vi "Update Tree.vi"(7 "Tree":refnum<vi>, 8 "error in (no error)":errorcluster, 10 "Task Run Info":T1[](array[typedef])) -> (0 "error out":errorcluster)   [LabVIEW 2020, in "Volatus.lvlib" / "DebugGUI.lvclass"]
uses:
  DebugGUI.lvclass
  Task Run Info.ctl
  Task Hierarchy.ctl
  Task State.ctl
  DebugGUI.lvclass/DebugGUI.ctl
  Volatus.lvlib
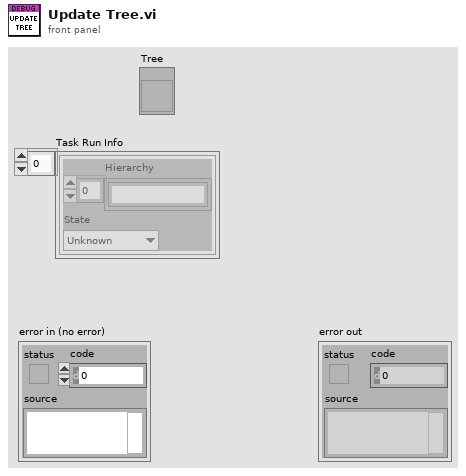
[diagram p1: front panel]
types:
  T1 = typedef "Volatus.lvlib/Task Run Info.ctl" = cluster{"Hierarchy":T2, "State":T3}
  T2 = typedef "Volatus.lvlib/Task Hierarchy.ctl" = string[]
  T3 = typedef "Volatus.lvlib/Task State.ctl" = enum16{"Unknown", "Idle", "Initializing", "Starting", "Running", "Stopping", "Stopped", "Error - Init", "Error - Start", "Error - Run", "Error - Stop"}
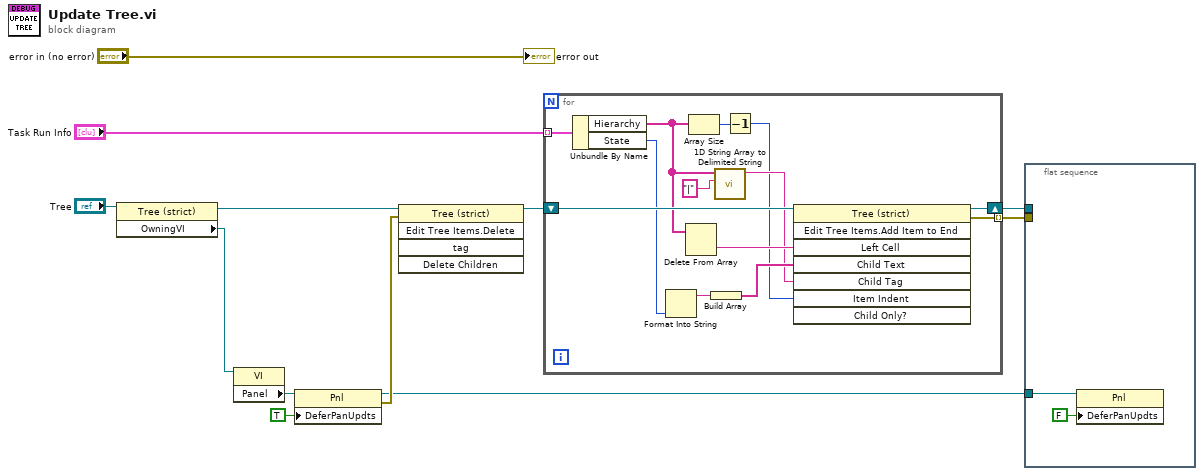
[diagram p0: block diagram]
diagram:
  n1 = property class="Tree (strict)"(reference="Tree") -> (reference out=w7:refnum<vi>, "OwningVI"=w10:refnum<vi>)  [unwired: 1 in, 1 out]
  n2 = property class="VI"(reference=w10) -> ("Panel"=w9:refnum<vi>)  [unwired: 1 in, 2 out]
  n3 = property class="Pnl"(reference=w9, "DeferPanUpdts"=TRUE ("Defer Panel Updates")) -> (reference out=w3:refnum<vi>, error out=w6:errorcluster)  [unwired: 1 in]
  n4 = invoke class="Tree (strict)" method="Edit Tree Items.Delete"(reference=w7, error in=w6) -> (reference out=w5:refnum<vi>)  [unwired: 3 in, 4 out]
  n5 = for {
    shift-right: [w15] -> w2
    shift-left: w5 -> [w25]
    tunnel: "Task Run Info" -> [w24] mode=indexing
    tunnel: [w14] -> w1 mode=indexing
    n6 = Unbundle By Name(w24) -> ("Hierarchy"=w18:T2, "State"=w23:T3)
    n7 = Format Into String(w23) -> (resulting string=w22:string)  [unwired: 3 in, 1 out]
    n8 = Delete From Array(array=w18) -> (deleted portion=w20:string)  [unwired: 2 in, 1 out]
    n9 = Array Size(array=w18) -> (size(s)=w19:i32)
    n10 = Build Array(w22) -> (w21:string[])
    n11 = call <vilib>:"1D String Array to Delimited String.vi"("delimiter"="|", "string array"=w18) -> ("delimited string"=w16:string)  [unwired: 9 in]
    n12 = Decrement(x=w19) -> (x-1=w13:i32)
    n13 = invoke class="Tree (strict)" method="Edit Tree Items.Add Item to End"(reference=w25, "Left Cell"=w20, "Child Text"=w21, "Child Tag"=w16, "Item Indent"=w13) -> (reference out=w15:refnum<vi>, error out=w14:errorcluster)  [unwired: 3 in, 6 out]
  }
  n14 = flat-sequence {
    tunnel: w3 -> [w26]
    tunnel: w2 -> [_]
    tunnel: w1 -> [_]
    frame #0 {
      n15 = property class="Pnl"(reference=w26, "DeferPanUpdts"=FALSE ("Defer Panel Updates")) -> ()  [unwired: 1 in, 2 out]
    }
  }
  "error out" <- "error in (no error)"
